vi "Stop Core.vi"(10 "final error code":i32, 11 "Results in":refnum<class "Results.lvclass">) -> (3 "Results out":refnum<class "Results.lvclass">)   [LabVIEW 2017, in "Result Actor.lvlib" / "Results.lvclass"]
uses:
  Results.lvclass
  Results.lvclass/Results.ctl
  <vilib>/ActorFramework/Actor/Actor.lvclass
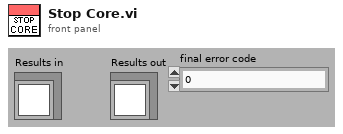
[diagram p1: front panel]
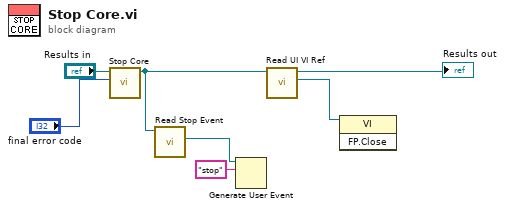
[diagram p0: block diagram]
diagram:
  n1 = call-parent "Stop Core.vi"("final error code"="final error code", "Actor in"="Results in") -> ("Actor out"=w3:refnum<class "Results.lvclass">)  [unwired: 9 in]
  n2 = call "Read Stop Event.vi"("Results in"=w3) -> ("stop event"=w6:refnum<user-event>)  [unwired: 8 in, 2 out]
  n3 = Generate User Event(user event=w6, event data cluster="stop" ("event data")) -> ()  [unwired: 2 in, 2 out]
  n4 = call "Read UI VI Ref.vi"("Results in"=w3) -> ("UI VI Ref"=w1:refnum<vi>, "Results out"=→"Results out":refnum<class "Results.lvclass">)  [unwired: 8 in, 1 out]
  n5 = invoke class="VI" method="FP.Close"(reference=w1) -> ()  [unwired: 2 in, 3 out]
